vi "Main.vi"() -> ()   [LabVIEW 2020]
uses:
  <vilib>/Utility/miscctls.llb/LVRectTypeDef.ctl
  Libraries/Determine Clicked Array Element Index/Determine Clicked Array Element Index.lvlib
  <vilib>/Dataflow_G/G-Audio/G-Audio.lvlib
  <vilib>/Dataflow_G/G-Audio/Controls/Audio Device Format.ctl
  <vilib>/Dataflow_G/G-Audio/Controls/Audio Device Config.ctl
  <vilib>/Dataflow_G/G-Audio/Audio Files/Polymorphic VIs/Open Audio File Read (Path).vi
  <vilib>/Dataflow_G/G-Audio/Controls/Audio File Refnum.ctl
  6933e24e-4767-4ff9-a2a1-095bcb724796.vi
  8390d630-45c6-4fd6-b59e-9795a7a5c185.vi
panel:
  in  "Stop Playing":bool
  out "Categories":string[](array[string])
  out "Sounds":string[][](array[string])
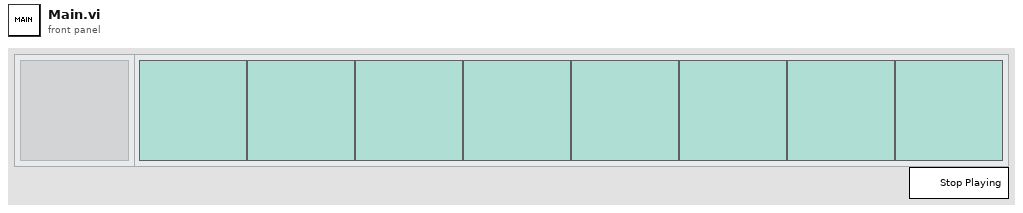
[diagram p1: front panel]
types:
  T1 = enum8{"Enabled", "Disabled", "Disabled and Grayed Out"}
  T2 = typedef "G-Audio.lvlib/Audio File Refnum.ctl" = refnum<file>
  T3 = typedef "LVRectTypeDef.ctl" = cluster{"Left":i16, "Top":i16, "Right":i16, "Bottom":i16}
  T4 = typedef "G-Audio.lvlib/Audio Device Config.ctl" = cluster{"Sample Rate (Hz)":u32, "Channels":u32, "Format":T5}
  T5 = typedef "G-Audio.lvlib/Audio Device Format.ctl" = enum16{"Native", "U8", "I16", "I32", "SGL"}
  T6 = typedef "G-Audio.lvlib/Audio Device Refnum.ctl" = refnum<file>
  T7 = typedef "LVPoint32TypeDef.ctl" = cluster{"Horizontal":i32, "Vertical":i32}
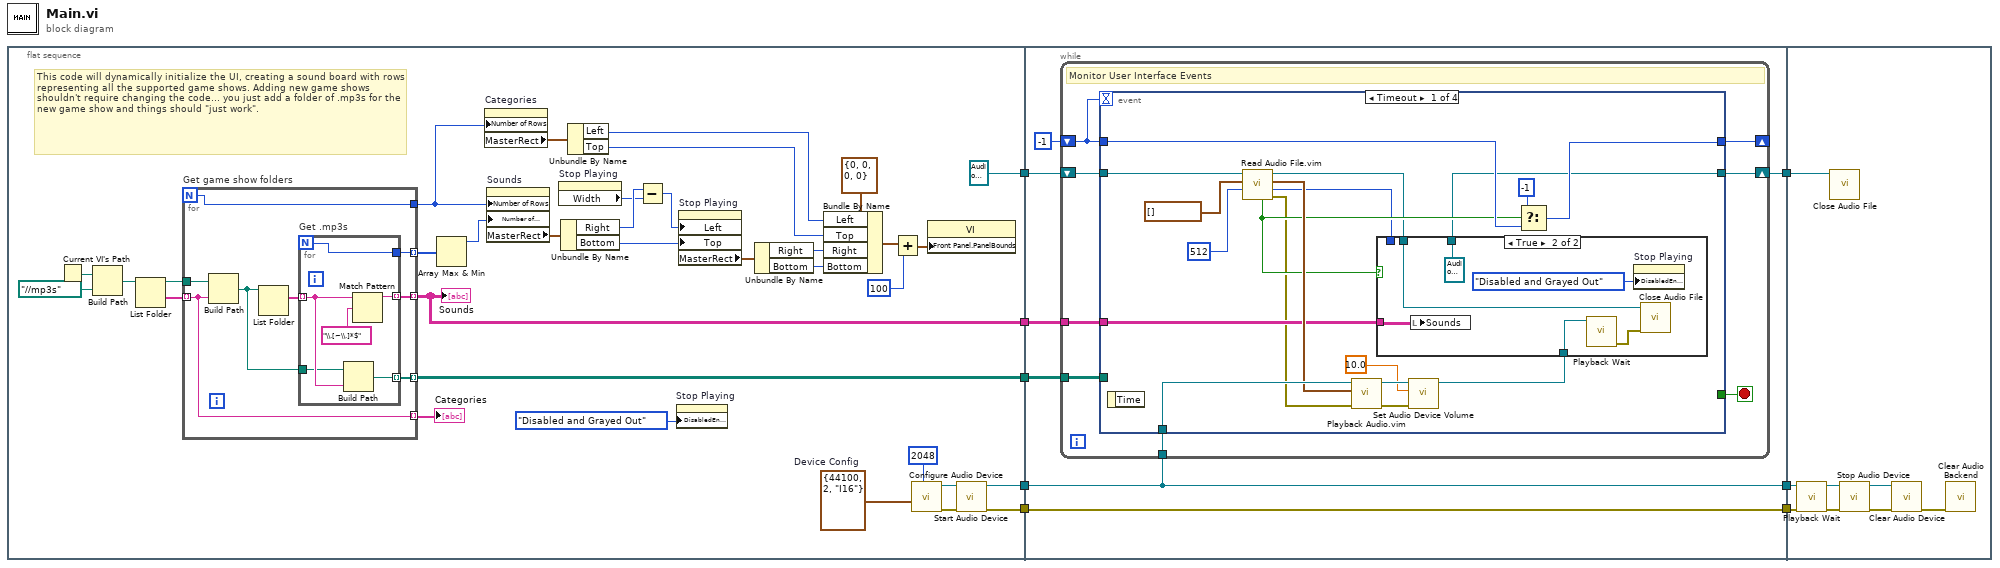
[diagram p0: block diagram]
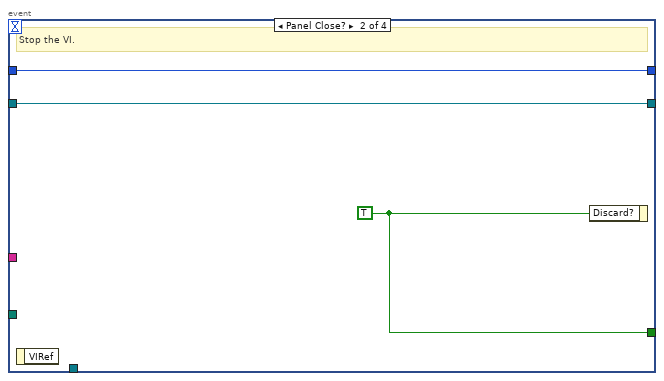
[diagram p3: hidden frame]
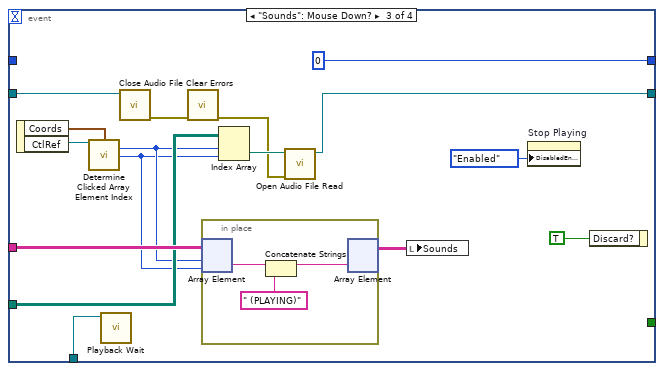
[diagram p4: hidden frame]
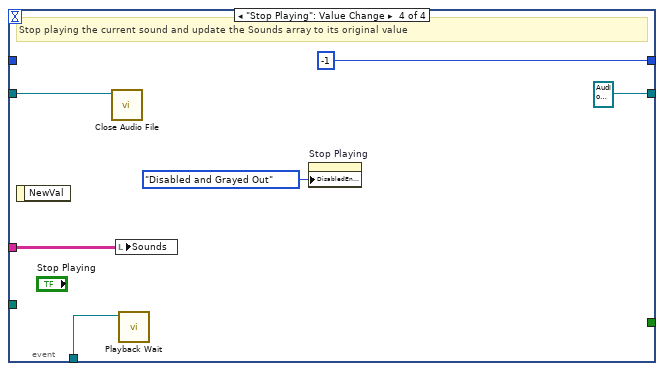
[diagram p5: hidden frame]
diagram:
  n1 = flat-sequence {
    tunnel: [w18] -> w8
    tunnel: [w17] -> w7
    tunnel: [w12] -> w5
    tunnel: [w11] -> w4
    tunnel: [T2 refnum ("Audio File Refnum")] -> w2
    tunnel: w8 -> [w62]
    tunnel: w7 -> [w61]
    tunnel: [w60] -> w6
    tunnel: w5 -> [w60]
    tunnel: w4 -> [w59]
    tunnel: [w59] -> w3
    tunnel: w2 -> [w58]
    tunnel: [w57] -> w1
    tunnel: w6 -> [w125]
    tunnel: w3 -> [w127]
    tunnel: w1 -> [w129]
    frame #0 {
      w14 = T4 {"Sample Rate (Hz)"=44100, "Channels"=2, "Format"=enum."I16"}  # Device Config
      # "This code will dynamically initialize the UI, creating a sound board with rows representing all the supported game shows. Adding new game shows shouldn't require changing the code... you just add a folder of .mp3s for the new game show and things should \"just work\"."
      n2 = Current VI's Path() -> (path=w41:path)
      n3 = Build Path(base path=w41, name or relative path=path "../../mp3s") -> (appended path=w42:path)
      n4 = List Folder(path=w42) -> (path out=w38:path, folder names=w39:string[])  [unwired: 3 in, 2 out]
      n5 = for "Get game show folders" {
        N -> [w46]
        tunnel: w39 -> [w49] mode=indexing
        tunnel: w38 -> [w50]
        tunnel: [w49] -> w37 mode=indexing
        tunnel: [w47] -> w17 mode=indexing
        tunnel: [w46] -> w36
        tunnel: [w45] -> w35 mode=indexing
        tunnel: [w43] -> w18 mode=indexing
        n6 = Build Path(base path=w50, name or relative path=w49) -> (appended path=w44:path)
        n7 = List Folder(path=w44) -> (filenames=w48:string[])  [unwired: 3 in, 3 out]
        n8 = for "Get .mp3s" {
          N -> [w54]
          tunnel: w48 -> [w53] mode=indexing
          tunnel: [w55] -> w47 mode=indexing
          tunnel: [w54] -> w45
          tunnel: w44 -> [w52]
          tunnel: [w51] -> w43 mode=indexing
          n9 = Build Path(base path=w52, name or relative path=w53) -> (appended path=w51:path)
          n10 = Match Pattern(string=w53, regular expression="\\.[~\\.]*$") -> (before substring=w55:string)  [unwired: 4 out]
        }
      }
      "Categories" <- w37
      "Sounds" <- w17
      n11 = Array Max & Min(array=w35) -> (max value=w34:i32)  [unwired: 3 out]
      n12 = property on="Categories" class="Arr (strict)"("Number of Rows"=w36) -> ("MasterRect"=w25:T3)  [unwired: 2 in, 2 out]
      n13 = property on="Sounds" class="Arr (strict)"("Number of Rows"=w36, "Number of Columns"=w34) -> ("MasterRect"=w33:T3)  [unwired: 2 in, 2 out]
      n14 = property on="Stop Playing" class="Bool"() -> ("Width"=w31:u32)  [unwired: 2 in, 2 out]
      n15 = Unbundle By Name(w33) -> ("Right"=w32:i16, "Bottom"=w29:i16)
      n16 = Unbundle By Name(w25) -> ("Left"=w24:i16, "Top"=w23:i16)
      n17 = Subtract(x=w32, y=w31) -> (x-y=w30:u32)
      n18 = property on="Stop Playing" class="Bool"("DisabledEnum"=T1."Disabled and Grayed Out" ("Disabled")) -> ()  [unwired: 2 in, 2 out]
      n19 = property on="Stop Playing" class="Bool"("Left"=w30, "Top"=w29) -> ("MasterRect"=w28:T3)  [unwired: 2 in, 2 out]
      n20 = Unbundle By Name(w28) -> ("Right"=w22:i16, "Bottom"=w21:i16)
      n21 = Bundle By Name(cluster=T3 {"Left"=0, "Top"=0, "Right"=0, "Bottom"=0} ("Front Panel Window:Panel Bounds"), "Left"=w24, "Top"=w23, "Right"=w22, "Bottom"=w21) -> (w26:T3)
      n22 = Add(x=w26, y=i16 100) -> (x+y=w20:T3)
      n23 = call <vilib>:"Configure Audio Device.vi"("Buffer Size (4096)"=2048 ("number of samples/ch"), "Device Config"=w14) -> ("error out"=w16:errorcluster, "Audio Device Refnum"=w15:T6)  [unwired: 6 in, 2 out]
      n24 = property class="VI"("Front Panel.PanelBounds"=w20) -> ()  [unwired: 2 in, 2 out]
      n25 = call <vilib>:"Start Audio Device.vi"("error in (no error)"=w16, "Audio Device Refnum In"=w15) -> ("error out"=w12:errorcluster, "Audio Device Refnum Out"=w11:T6)  [unwired: 8 in]
    }
    frame #1 {
      n26 = while {
        shift-right: [w69] -> _
        shift-left: -1 -> [w70]
        tunnel: w62 -> [w68]
        tunnel: w61 -> [w67]
        tunnel: w59 -> [w66]
        shift-right: [w65] -> w57
        shift-left: w58 -> [w64]
        stop <- w71 stop-if-true
        # "Monitor User Interface Events"
        n27 = event shown="[0] Timeout" {
          selector: _ -> [_ _ _ _]
          dyn-events: _ -> [_ _ _ _]
          timeout: w70 -> [_ _ _ _]
          tunnel: [_ w99 _ _] -> w71
          tunnel: w70 -> [w85 w98 _ _]
          tunnel: [w86 w98 0 -1] -> w69
          tunnel: w68 -> [_ _ w110 _]
          tunnel: w67 -> [w77 _ w112 w124]
          tunnel: w66 -> [w83 _ w101 w120]
          tunnel: [w74 w97 w106 T2 refnum ("Audio File Refnum")] -> w65
          tunnel: w64 -> [w89 w97 w105 w122]
          event Timeout {
            n28 = event-data() -> ()  [unwired: 1 in, 1 out]
            n29 = call "Read Audio File.vim"("Frames To Read"=u64 512, "Data Format"=waveform(i16)[] [], "Audio File Refnum In"=w89) -> ("error out"=w76:errorcluster, "Frames Read"=w72:u64, "Audio Data"=w82:waveform(i16)[], "Audio File Refnum Out"=w75:T2, "End of File?"=w78:bool)  [unwired: 4 in]
            n30 = call "Playback Audio.vim"("error in (no error)"=w76, "Audio Data"=w82, "Audio Device Refnum In"=w83) -> ("error out"=w80:errorcluster, "Audio Device Refnum Out"=w81:T6)  [unwired: 7 in]
            n31 = call <vilib>:"Set Audio Device Volume.vi"("error in (no error)"=w80, "Volume"=sgl 10.0, "Audio Device Refnum In"=w81) -> ("Audio Device Refnum Out"=w73:T6)  [unwired: 7 in, 1 out]
            n32 = case shown="True" w78 {
              tunnel: w77 -> [_ w96]
              tunnel: w75 -> [w90 w95]
              tunnel: [w90 T2 refnum ("Audio File Refnum")] -> w74
              tunnel: w73 -> [_ w93]
              tunnel: w72 -> [_ _]
              frame False {
              }
              frame True {
                n33 = local write "Sounds"(w96) -> ()
                n34 = call <vilib>:"Playback Wait.vi"("Audio Device Refnum In"=w93) -> ("error out"=w92:errorcluster)  [unwired: 9 in, 1 out]
                n35 = property on="Stop Playing" class="Bool"("DisabledEnum"=T1."Disabled and Grayed Out" ("Disabled")) -> ()  [unwired: 2 in, 2 out]
                n36 = call <vilib>:"Close Audio File.vi"("error in (no error)"=w92, "Audio File Refnum In"=w95) -> ()  [unwired: 9 in, 1 out]
              }
            }
            n37 = Select(t=-1, s=w78, f=w85) -> (s? t:f=w86:i32)
          }
          event Panel Close? {
            w99 = TRUE ("Discard?")
            # "Stop the VI."
            n38 = event-data() -> ()  [unwired: 1 in, 1 out]
            n39 = event-data("Discard?"=w99) -> ()  [unwired: 1 in, 1 out]
          }
          event "Sounds": Mouse Down? {
            n40 = event-data() -> ("Coords"=w114:T7, "CtlRef"=w115:refnum<vi>)  [unwired: 1 in]
            n41 = call "Determine Clicked Array Element Index.vi"("reference"=w115, "Coords of Click"=w114) -> ("Clicked Row"=w109:i32, "Clicked Col"=w108:i32)  [unwired: 8 in, 4 out]
            n42 = call <vilib>:"Playback Wait.vi"("Audio Device Refnum In"=w101) -> ()  [unwired: 9 in, 2 out]
            n43 = call <vilib>:"Close Audio File.vi"("Audio File Refnum In"=w105) -> ("error out"=w104:errorcluster)  [unwired: 10 in]
            n44 = call <vilib>:"Clear Errors.vi"("error in (no error)"=w104) -> ("error out"=w103:errorcluster)  [unwired: 5 in, 1 out]
            n45 = in-place {
              n46 = in-place-array #1(w112, w109, w108) -> (w118:string)
              n47 = Concatenate Strings(w118, " (PLAYING)") -> (w117:string)
              n48 = in-place-array #1(w117) -> (w111:string[][])  [unwired: 2 out]
            }
            n49 = Index Array(array=w110, index (row)=w109, index (col)=w108) -> (element=w107:path)
            n50 = call-poly <vilib>:"Open Audio File Read.vi"("error in (no error)"=w103, "Path"=w107) -> ("Audio File Refnum"=w106:T2)  [unwired: 8 in, 1 out]
            n51 = local write "Sounds"(w111) -> ()
            n52 = property on="Stop Playing" class="Bool"("DisabledEnum"=T1."Enabled" ("Disabled")) -> ()  [unwired: 2 in, 2 out]
            n53 = event-data("Discard?"=TRUE) -> ()  [unwired: 1 in, 1 out]
          }
          event "Stop Playing": Value Change {
            # "Stop playing the current sound and update the Sounds array to its original value"
            n54 = event-data() -> ()  [unwired: 1 in, 1 out]
            n55 = call <vilib>:"Close Audio File.vi"("Audio File Refnum In"=w122) -> ()  [unwired: 10 in, 1 out]
            n56 = local write "Sounds"(w124) -> ()
            n57 = call <vilib>:"Playback Wait.vi"("Audio Device Refnum In"=w120) -> ()  [unwired: 9 in, 2 out]
            n58 = property on="Stop Playing" class="Bool"("DisabledEnum"=T1."Disabled and Grayed Out" ("Disabled")) -> ()  [unwired: 2 in, 2 out]
          }
        }
      }
    }
    frame #2 {
      n59 = call <vilib>:"Playback Wait.vi"("error in (no error)"=w125, "Audio Device Refnum In"=w127) -> ("error out"=w126:errorcluster, "Audio Device Refnum Out"=w128:T6)  [unwired: 8 in]
      n60 = call <vilib>:"Close Audio File.vi"("Audio File Refnum In"=w129) -> ()  [unwired: 10 in, 1 out]
      n61 = call <vilib>:"Stop Audio Device.vi"("error in (no error)"=w126, "Audio Device Refnum In"=w128) -> ("error out"=w131:errorcluster, "Audio Device Refnum Out"=w132:T6)  [unwired: 8 in]
      n62 = call <vilib>:"Clear Audio Device.vi"("error in (no error)"=w131, "Audio Device Refnum In"=w132) -> ("error out"=w130:errorcluster)  [unwired: 9 in]
      n63 = call <vilib>:"Clear Audio Backend.vi"("error in (no error)"=w130) -> ()  [unwired: 10 in, 1 out]
    }
  }
